vi "Split TargetPanel by Node.vi"(6 "VI*":refnum<vi>, 8 "error in":errorcluster caption="错误输入（无错误）", 9 "Split Mode":T1, 10 "Node*":refnum<data-value>, 11 "PCM PanelSplit in":refnum<class "PCM PanelSplit.lvclass"> caption="DNL_LabVIEW Object in") -> (0 "error out":errorcluster caption="错误输出", 2 "ChildDataNode[]":refnum<data-value>[](array[refnum]), 3 "PCM PanelSplit out":refnum<class "PCM PanelSplit.lvclass"> caption="DNL_LabVIEW Object out")   [LabVIEW 2016, in "PCM PanelSplit.lvclass"]
uses:
  PCM PanelSplit.lvclass
  PanelSplitToolkit/PanelObject/PanelObject.lvclass
  PanelSplitToolkit/PanelDataNode/Split Mode.ctl
  PanelSplitToolkit/PanelDataNode/PanelDataNode.lvclass
  PanelSplitToolkit/PanelRootNode/PanelRootNode.lvclass
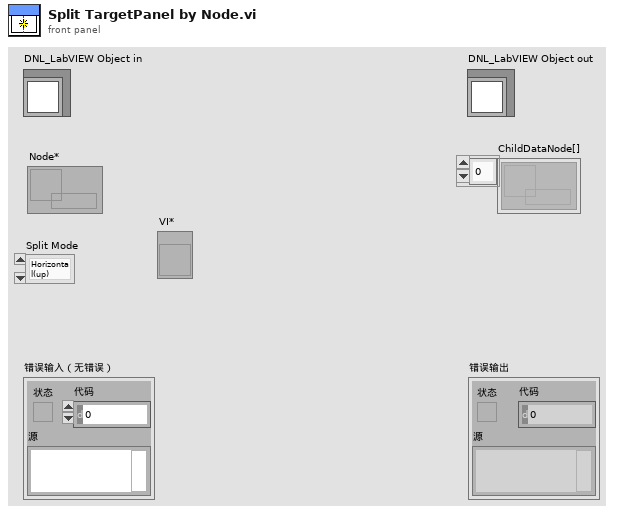
[diagram p1: front panel]
types:
  T1 = typedef "PanelDataNode.lvclass/Split Mode.ctl" = enum16{"Horizontal(up)", "Vertical(left)", "Horizontal(down)", "Vertical(right)"}
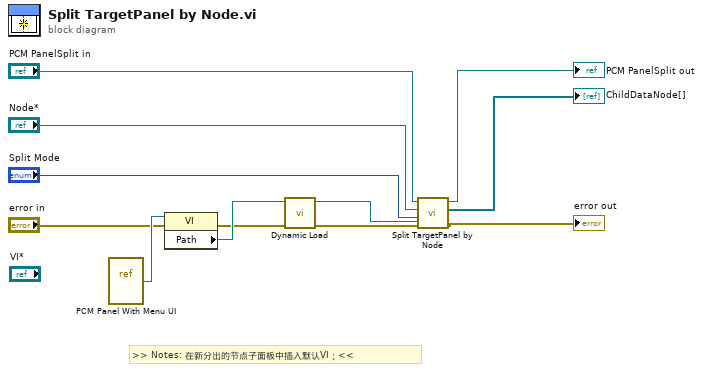
[diagram p0: block diagram]
diagram:
  # ">> Notes: 在新分出的节点子面板中插入默认VI；<<"
  n1 = vi-ref "PCM Panel With Menu UI.vi"() -> (w9:refnum<vi>)
  n2 = property class="VI"(reference=w9, error in="error in") -> (error out=w2:errorcluster, "Path"=w8:path)  [unwired: 1 out]
  n3 = call "Dynamic Load.vi"("error in"=w2, "Vi Path"=w8) -> ("错误输出"=w1:errorcluster, "vi reference"=w5:refnum<vi>)  [unwired: 8 in]
  n4 = call-parent "Split TargetPanel by Node.vi"("Dynamic VI*"=w5, "error in"=w1, "Split Mode"="Split Mode", "Node*"="Node*", "PanelRootNode 输入"="PCM PanelSplit in") -> ("error out"=→"error out":errorcluster, "ChildDataNode[]"=→"ChildDataNode[]":refnum<data-value>[], "PanelRootNode 输出"=→"PCM PanelSplit out":refnum<class "PCM PanelSplit.lvclass">)  [unwired: 4 in]
